vi "Read.vi"(8 "error in (no error)":errorcluster, 11 "NiPxi6123 in":refnum<class "NiPxi6123.lvclass">) -> (0 "error out":errorcluster, 3 "NiPxi6123 out":refnum<class "NiPxi6123.lvclass">)   [LabVIEW 2014, in "SamplerPlugins.lvlib" / "NiPxi6123.lvclass"]
uses:
  NiPxi6123.lvclass
  <vilib>/DAQmx/read.llb/DAQmx Read (Analog 1D DBL NChan 1Samp).vi
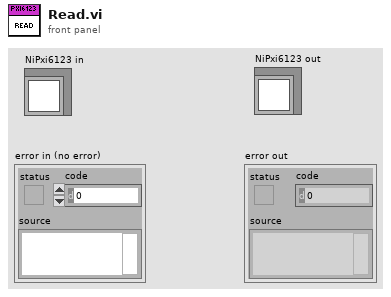
[diagram p1: front panel]
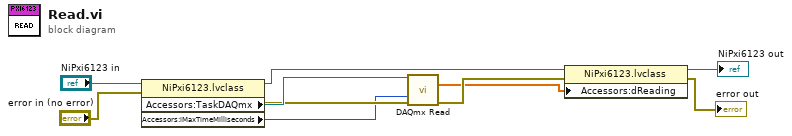
[diagram p0: block diagram]
diagram:
  n1 = property class="NiPxi6123.lvclass"(reference="NiPxi6123 in", error in="error in (no error)") -> (reference out=w5:refnum<class "NiPxi6123.lvclass">, error out=w7:errorcluster, "Accessors:TaskDAQmx"=w8:refnum<k21>, "Accessors:iMaxTimeMilliseconds"=w6:i32)
  n2 = call-poly <vilib>:"DAQmx Read.vi"("task/channels in"=w8, "timeout"=w6, "error in"=w7) -> ("data"=w1:dbl[], "error out"=w4:errorcluster)  [unwired: 10 in, 1 out]
  n3 = property class="NiPxi6123.lvclass"(reference=w5, error in=w4, "Accessors:dReading"=w1) -> (reference out=→"NiPxi6123 out":refnum<class "NiPxi6123.lvclass">, error out=→"error out":errorcluster)
